vi "PH_Timing.evt call set Slow Trigger.vi"(0 "i ref in":refnum<vi>, 2 "Instance":string, 3 "Slow Trigger Settings":T1, 5 "error in (no error)":errorcluster) -> (14 "i ref out":refnum<vi>, 19 "error out":errorcluster)   [LabVIEW 2014, in "PH_Timing.lvlib"]
doc: "This VI calls the case \"SlowTrig\" by a simple call."
uses:
  PH_Timing.lvlib
  PH_Timing.Slow Trigger Settings.ctl
  CS_Core/CSSystem/CoreLib/CoreLib.short 2 byte array.vi
  CS_Core/CSSystem/CoreLib/CoreLib.double 2 byte array.vi
  CS_Core/BaseProcess/BaseProcess.lvlib
  CS_Core/CSSystem/CoreLib/CoreLib.lvlib
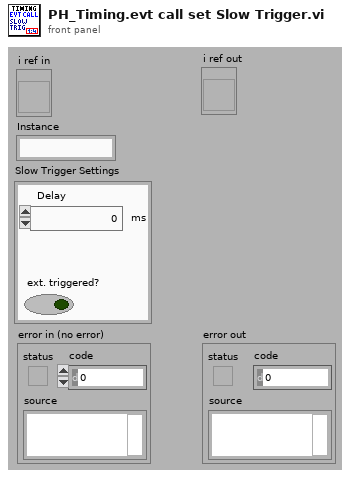
[diagram p1: front panel]
types:
  T1 = typedef "PH_Timing.lvlib/PH_Timing.Slow Trigger Settings.ctl" = cluster{"Delay":dbl, "externally triggered?":bool}
  T2 = typedef "CoreDefs.rawDataType.ctl" = i8[]
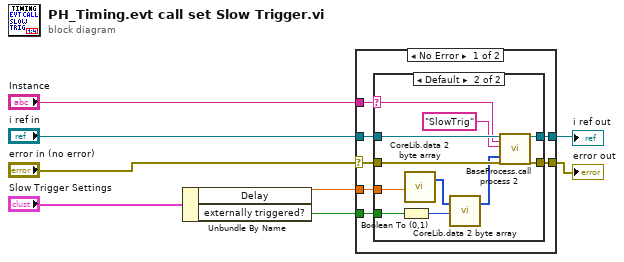
[diagram p0: block diagram]
diagram:
  n1 = Unbundle By Name("Slow Trigger Settings") -> ("Delay"=w2:dbl, "externally triggered?"=w1:bool)
  n2 = case shown="No Error" "error in (no error)" {
    selector: "error in (no error)" -> [w11 w29]
    tunnel: [w15 w30] -> w5
    tunnel: [w14 w29] -> w4
    tunnel: "i ref in" -> [w13 w30]
    tunnel: "Instance" -> [w12 _]
    tunnel: w2 -> [w10 _]
    tunnel: w1 -> [w9 _]
    frame No Error {
      n3 = case shown="Default" w12 {
        selector: w12 -> [_ w23]
        tunnel: [w17 w28] -> w15
        tunnel: [w16 w27] -> w14
        tunnel: w13 -> [w17 w26]
        tunnel: w11 -> [w16 w25]
        tunnel: w10 -> [_ w22]
        tunnel: w9 -> [_ w19]
        frame "N/A" {
        }
        frame Default {
          n4 = Boolean To (0,1)(Boolean=w19) -> (0, 1=w18:i16)
          n5 = call-poly "CoreLib.data 2 byte array.vi"("f64"=w22) -> ("byteArray out"=w21:T2)  [unwired: 18 in]
          n6 = call-poly "CoreLib.data 2 byte array.vi"("byteArray"=w21, "i16"=w18) -> ("byteArray out"=w20:T2)  [unwired: 17 in]
          n7 = call "BaseProcess.call process 2.vi"("i ref in"=w26, "Object"=w23, "Selector"="SlowTrig", "Data"=w20, "error in (no error)"=w25) -> ("i ref out"=w28:refnum<vi>, "error out"=w27:errorcluster)  [unwired: 13 in]
        }
      }
    }
    frame Error {
    }
  }
  "error out" <- w4
  "i ref out" <- w5
